vi "APS get axis info.vi"(0 "Axis_ID":i32, 1 "Module_ID":i32, 5 "Board_ID":i32, 7 "Axis_No":i32, 9 "Port_ID":i32, 11 "error in (no error)":errorcluster caption="错误输入（无错误）") -> (3 "Module_ID out":i32, 4 "function return":i32, 6 "Board_ID out":i32, 8 "Axis_No out":i32, 10 "Port_ID out":i32, 15 "error out":errorcluster caption="错误输出")   [LabVIEW 2011, in "APS168.lvlib"]
doc: "I32 FNTYPE APS_get_axis_info( I32 Axis_ID, I32 *Board_ID, I32 *Axis_No, I32 *Port_ID, I32 *Module_ID );"
uses:
  APS168.lvlib
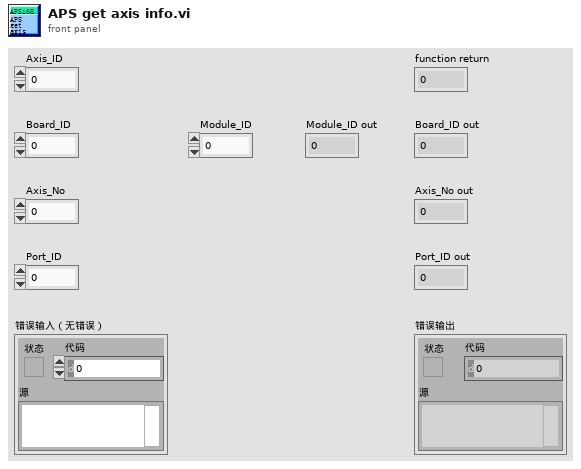
[diagram p1: front panel]
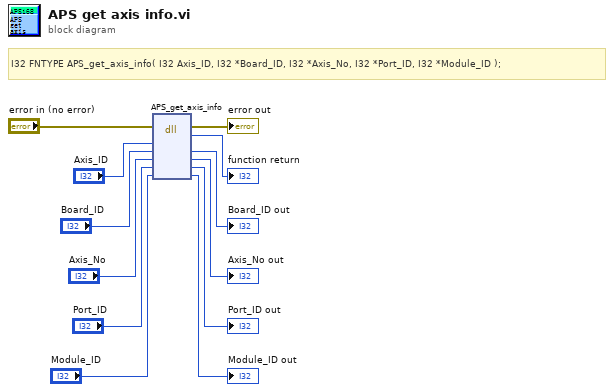
[diagram p0: block diagram]
diagram:
  # "I32 FNTYPE APS_get_axis_info( I32 Axis_ID, I32 *Board_ID, I32 *Axis_No, I32 *Port_ID, I32 *Module_ID );"
  n1 = dll-call lib="PTH1Labs E软件ADLINK 204CAPS_1_7_1_LIB line 连续运动204APS168.*" fn="APS_get_axis_info"(error in="error in (no error)", "Axis_ID"="Axis_ID", "Board_ID"="Board_ID", "Axis_No"="Axis_No", "Port_ID"="Port_ID", "Module_ID"="Module_ID") -> (error out=→"error out":errorcluster, →"function return":i32, "Board_ID"=→"Board_ID out":i32, "Axis_No"=→"Axis_No out":i32, "Port_ID"=→"Port_ID out":i32, "Module_ID"=→"Module_ID out":i32)  [unwired: 3 in, 1 out]
